vi "StopWalkabout.vi"(0 "reference in":refnum<class "Object.lvclass">, 2 "ms timeout (-1)":i32=-1, 5 "error in (no error)":errorcluster) -> (14 "reference out":refnum<class "Object.lvclass">, 19 "error out":errorcluster)   [LabVIEW 2020, in "Object.lvclass"]
uses:
  Object.lvclass
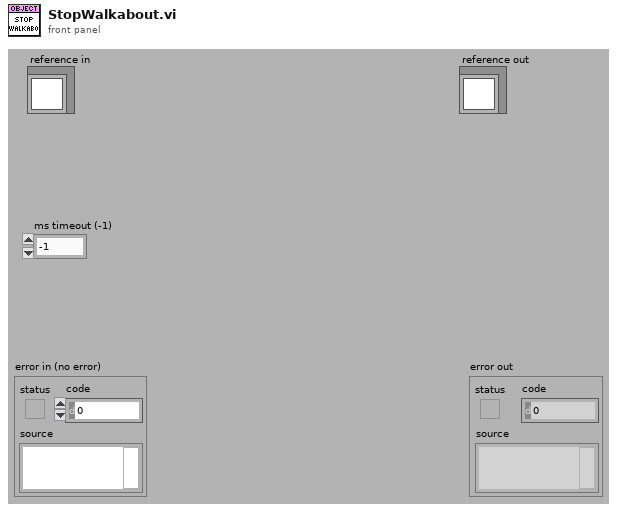
[diagram p1: front panel]
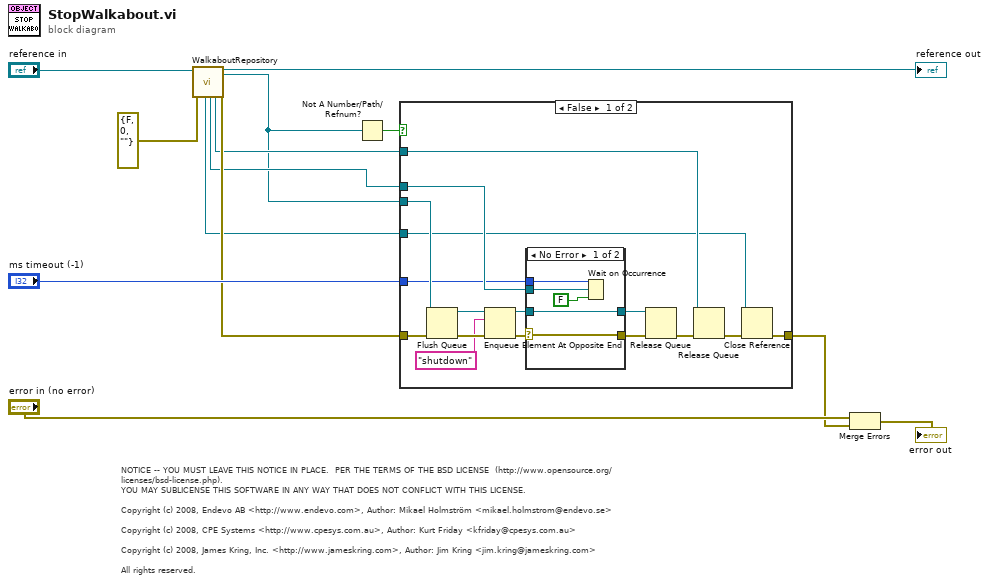
[diagram p0: block diagram]
diagram:
  # "NOTICE -- YOU MUST LEAVE THIS NOTICE IN PLACE.  PER THE TERMS OF THE BSD LICENSE  (http://www.opensource.org/licenses/bsd-license.php).\nYOU MAY SUBLICENSE THIS SOFTWARE IN ANY WAY THAT DOES NOT CONFLICT WITH THIS LICENSE.\n\nCopyright (c) 2008, Endevo AB <http://www.endevo.com>, Author: Mikael Holmström <mikael.holmstrom@endevo.se>\n\nCopyright (c) 2008, CPE Systems <http://www.cpesys.com.au>, Author: Kurt Friday <kfriday@cpesys.com.au>\n\nCopyright (c) 2008, James Kring, Inc. <http://www.jameskring.com>, Author: Jim Kring <jim.kring@jameskring.com>\n\nAll rights reserved."
  n1 = call "WalkaboutRepository.vi"("reference in"="reference in", "error in (no error)"=errorcluster {"status"=FALSE, "code"=0, "source"=""}) -> ("ProcessViRef"=w4:refnum<vi>, "ProcessSyncOccurrence"=w6:refnum<k4>, "FromProcessQueue"=w5:refnum<queue>, "reference out"=→"reference out":refnum<class "Object.lvclass">, "ToProcessQueue"=w2:refnum<queue>, "error out"=w7:errorcluster)  [unwired: 12 out]
  n2 = Not A Number/Path/Refnum?(number/path/refnum=w2) -> (NaN/Path/Refnum?=w1:bool)
  n3 = case shown="False" w1 {
    tunnel: w6 -> [w24 _]
    tunnel: w7 -> [w26 w37]
    tunnel: [w18 w37] -> w11
    tunnel: w2 -> [w29 _]
    tunnel: "ms timeout (-1)" -> [w17 _]
    tunnel: w5 -> [w15 _]
    tunnel: w4 -> [w14 _]
    frame False {
      n4 = Flush Queue(queue=w29, error in (no error)=w26) -> (queue out=w27:refnum<queue>, error out=w28:errorcluster)  [unwired: 1 out]
      n5 = Enqueue Element At Opposite End(queue=w27, element="shutdown", error in (no error)=w28) -> (queue out=w23:refnum<queue>, error out=w16:errorcluster)  [unwired: 2 out]
      n6 = case shown="No Error" w16 {
        tunnel: [w30 w36] -> w22
        tunnel: w24 -> [w34 _]
        tunnel: [w32 w35] -> w21
        tunnel: w23 -> [w32 w35]
        tunnel: w17 -> [w31 _]
        selector: w16 -> [w30 w36]
        frame No Error {
          n7 = Wait on Occurrence(1:FALSE ("ignore previous (T)"), 2:w34, 3:w31) -> ()  [unwired: 1 out]
        }
        frame Error {
        }
      }
      n8 = Release Queue(queue=w21, error in (no error)=w22) -> (error out=w20:errorcluster)  [unwired: 3 out]
      n9 = Release Queue(queue=w15, error in (no error)=w20) -> (error out=w19:errorcluster)  [unwired: 3 out]
      n10 = Close Reference(reference=w14, error in (no error)=w19) -> (error out=w18:errorcluster)
    }
    frame True {
    }
  }
  n11 = Merge Errors("error in (no error)", w11) -> (→"error out":errorcluster)
